vi "recombine group data.vi"(8 "error in":errorcluster, 9 "specification":T1[](array[typedef]), 10 "group in":T3, 11 "data table in":T3) -> (0 "error out":errorcluster, 2 "group out":T3, 3 "data table out":T3)   [LabVIEW 2013, in "data bus values.lvlib"]
doc: "Accepts a primary data table and a subgroup data table, and copies data from the group into the main table."
uses:
  data bus values.lvlib
  data table.ctl
  group specification.ctl
  tag/Data Type.ctl
  data polymorphs/write many/write Doubles.vi
  data polymorphs/read all/read all Doubles.vi
  data polymorphs/write many/write I64s.vi
  data polymorphs/read all/read all I64s.vi
  data polymorphs/write many/write Booleans.vi
  data polymorphs/read all/read all Booleans.vi
  data polymorphs/write many/write Array of Doubles.vi
  data polymorphs/read all/read all Array of Doubles.vi
  data polymorphs/write many/write Array of I64s.vi
  data polymorphs/read all/read all Array of I64s.vi
  data polymorphs/write many/write Variants.vi
  data polymorphs/read all/read all Variants.vi
  tag/data bus tag description.lvclass
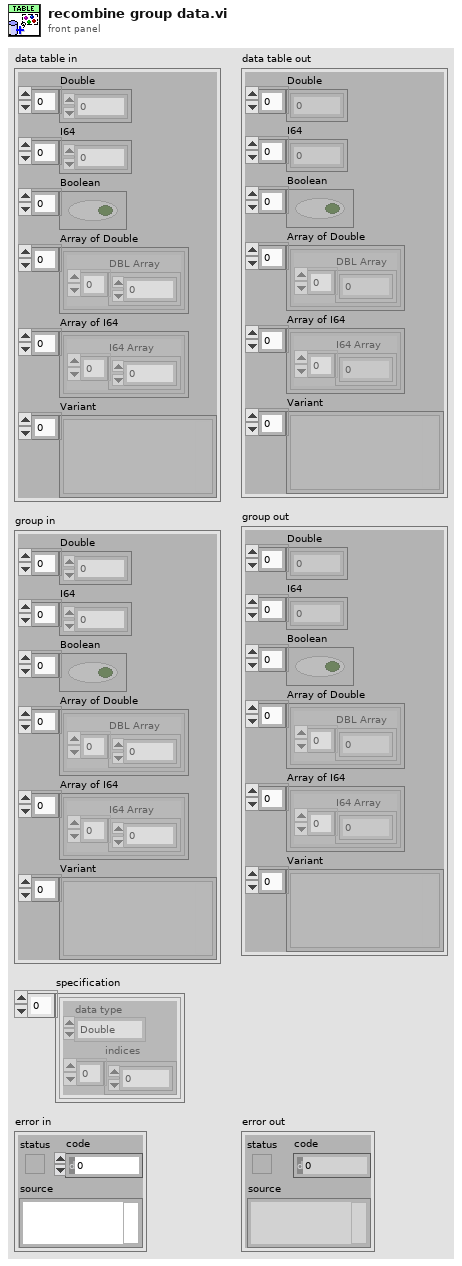
[diagram p1: front panel]
types:
  T1 = typedef "data bus values.lvlib/group specification.ctl" = cluster{"data type":T2, "indices":i32[]}
  T2 = typedef "data bus tag description.lvclass/Data Type.ctl" = enum16{"Double", "I64", "Boolean", "Array of Double", "Array of I64", "Variant"}
  T3 = typedef "data bus values.lvlib/data table.ctl" = cluster{"Double":dbl[], "I64":i64[], "Boolean":bool[], "Array of Double":cluster{"DBL Array":dbl[]}[], "Array of I64":cluster{"I64 Array":i64[]}[], "Variant":variant[]}
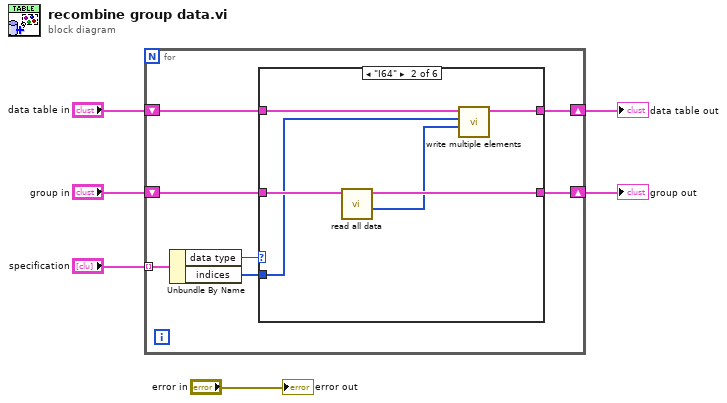
[diagram p0: block diagram]
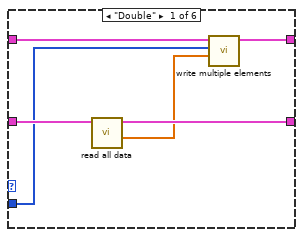
[diagram p2: hidden frame]
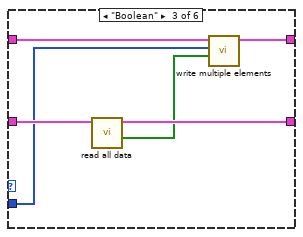
[diagram p3: hidden frame]
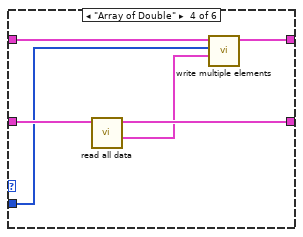
[diagram p4: hidden frame]
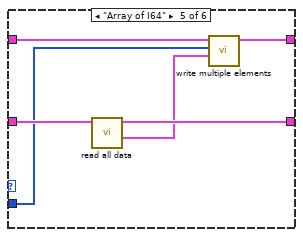
[diagram p5: hidden frame]
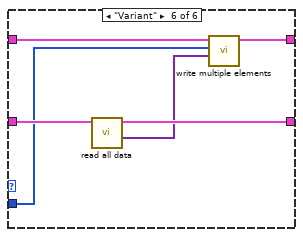
[diagram p6: hidden frame]
diagram:
  n1 = for {
    shift-right: [w9] -> w5
    shift-left: "data table in" -> [w10]
    shift-right: [w7] -> w3
    shift-left: "group in" -> [w8]
    tunnel: "specification" -> [w13] mode=indexing
    n2 = Unbundle By Name(w13) -> ("data type"=w12:T2, "indices"=w11:i32[])
    n3 = case shown="\"I64\"" w12 {
      tunnel: w11 -> [w14 w20 w26 w32 w38 w44]
      tunnel: w10 -> [w16 w22 w28 w34 w40 w46]
      tunnel: [w15 w21 w27 w33 w39 w45] -> w9
      tunnel: w8 -> [w19 w25 w31 w37 w43 w49]
      tunnel: [w18 w24 w30 w36 w42 w48] -> w7
      frame "Double" {
        n4 = call-poly "read all data.vi"("data table in"=w19) -> ("values"=w17:dbl[], "data table out"=w18:T3)  [unwired: 9 in]
        n5 = call-poly "write multiple elements.vi"("values"=w17, "indices"=w14, "data table in"=w16) -> ("data table out"=w15:T3)  [unwired: 8 in]
      }
      frame "I64" {
        n6 = call-poly "read all data.vi"("data table in"=w25) -> ("values"=w23:i64[], "data table out"=w24:T3)  [unwired: 9 in]
        n7 = call-poly "write multiple elements.vi"("values"=w23, "indices"=w20, "data table in"=w22) -> ("data table out"=w21:T3)  [unwired: 8 in]
      }
      frame "Boolean" {
        n8 = call-poly "read all data.vi"("data table in"=w31) -> ("values"=w29:bool[], "data table out"=w30:T3)  [unwired: 9 in]
        n9 = call-poly "write multiple elements.vi"("values"=w29, "indices"=w26, "data table in"=w28) -> ("data table out"=w27:T3)  [unwired: 8 in]
      }
      frame "Array of Double" {
        n10 = call-poly "read all data.vi"("data table in"=w37) -> ("values"=w35:cluster{"Array":dbl[]}[], "data table out"=w36:T3)  [unwired: 9 in]
        n11 = call-poly "write multiple elements.vi"("values"=w35, "indices"=w32, "data table in"=w34) -> ("data table out"=w33:T3)  [unwired: 8 in]
      }
      frame "Array of I64" {
        n12 = call-poly "read all data.vi"("data table in"=w43) -> ("values"=w41:cluster{"Array":i64[]}[], "data table out"=w42:T3)  [unwired: 9 in]
        n13 = call-poly "write multiple elements.vi"("values"=w41, "indices"=w38, "data table in"=w40) -> ("data table out"=w39:T3)  [unwired: 8 in]
      }
      frame "Variant" {
        n14 = call-poly "read all data.vi"("data table in"=w49) -> ("values"=w47:variant[], "data table out"=w48:T3)  [unwired: 9 in]
        n15 = call-poly "write multiple elements.vi"("values"=w47, "indices"=w44, "data table in"=w46) -> ("data table out"=w45:T3)  [unwired: 8 in]
      }
    }
  }
  "data table out" <- w5
  "group out" <- w3
  "error out" <- "error in"
